vi "Vision_Processing_R_R6.vi"(0 "Current State":T1(ring)=enum."Normal - 5", 1 "Image Dst":T6=refnum, 2 "Inpute Image":T6=refnum, 3 "Startup Flag":bool, 5 "Current ROI Descriptor":T11={"Global Rectangle"=[0, 0, 320, 240], "Contours"=[{"ID"=enum."External", "Type"=12, "Coordinates"=[0, 0, 320, 240, 0]}]} {"Contours"."Type" items=["No Selection", "Point", "Line", "Rectangle", "Oval", "Polygon", "Freehand Region", "Annulus", "Unused2", "Unused3", "Broken Line", "Freehand Line", "Rotated Rectangle"]}, 6 "Avg Score - Last":dbl=802.5034383138021, 7 "error in (no error)":errorcluster, 8 "Current Settings":T9={"Curve Parameters"={"Extraction Mode"=1, "Edge Threshold"=150, "Edge Filter Size"=0, "Min Length"=25, "Row Search Step Size"=15, "Col Search Step Size"=15, "Max Endpoint Gap"=2, "Closed"=TRUE, "Subpixel"=TRUE}, "Match Mode"={"Rotation"=TRUE, "Scale"=TRUE, "Occlusion"=TRUE, "Reserved"=FALSE, "Reserved"=FALSE, "Reserved"=FALSE}, "Range Settings"=[{"Match Constraints"=0, "Min"=-5.0, "Max"=5.0}, {"Match Constraints"=1, "Min"=20.0, "Max"=150.0}, {"Match Constraints"=2, "Min"=0.0, "Max"=25.0}], "Number of Matches"=1, "Minimum Match Score"=800.0, "SubPixel Accuracy"=TRUE, "Adv. Geometric Match Options 2"=[{"Setup Data Item"=20, "Item Value"=0.0}, {"Setup Data Item"=22, "Item Value"=1.0}]} {"Curve Parameters"."Extraction Mode" items=["Normal", "Uniform Regions"]; "Curve Parameters"."Edge Filter Size" items=["Fine", "Normal", "Contour Tracing"]; "Curve Parameters"."Max Endpoint Gap" min=0; "Curve Parameters"."Col Search Step Size" min=1 max=255 step=1; "Curve Parameters"."Row Search Step Size" min=1 max=255 step=1; "Curve Parameters"."Min Length" min=0; "Curve Parameters"."Edge Threshold" min=1 max=350 step=1; "Range Settings"."Max" format="%.2f"; "Range Settings"."Min" format="%.2f"; "Range Settings"."Match Constraints" items=["Rotation Angle (degrees)", "Scale Factor (%)", "Occlusion (%)"]; "Adv. Geometric Match Options 2"."Setup Data Item" items=["Curve Extraction Mode", "Curve Edge Threshold", "Curve Edge Filter Size", "Min Curve Length", "Curve Row Search Step Size", "Curve Col Search Step Size", "Curve Max Endpoint Gap", "Extract Closed Curves", "Enable Subpixel Curve Extraction", "Enable Correlation Score", "Enable Subpixel Accuracy", "Subpixel Iterations", "Subpixel Tolerance", "Initial Match List Length", "Enable Target Template Curve Score", "Min Match Separation Distance", "Min Match Separation Angle", "Min Match Separation Scale", "Max Match Overlap", "Enable Coarse Result", "Enable Calibration Support", "Enable Contrast Reversal", "Search Strategy", "Refinement Match Factor", "Subpixel Match Factor"]}, 9 "Sub Beacon Search Enable":bool[](array[boolean])=[FALSE, FALSE, FALSE, FALSE, FALSE], 10 "History Data - IN":T5={"Valid Beacon History - in"=[FALSE, FALSE, FALSE, FALSE, FALSE, FALSE, FALSE, FALSE, FALSE, FALSE, FALSE, FALSE, FALSE, FALSE, FALSE, FALSE, FALSE, FALSE, FALSE, FALSE], "Valid Score History"=[916.1194458007812, 0.0, 921.171142578125, 952.2998657226562, 947.6416015625, 946.7607421875, 946.6710815429688, 913.2891235351562, 946.3783569335938, 946.1008911132812, 949.7362060546875, 948.7965087890625, 947.1905517578125, 948.5363159179688, 949.03466796875, 951.10986328125, 800.9814453125, 952.3334350585938, 926.0540161132812, 946.85888671875], "Valid Scale History"=[77.35153198242188, 0.0, 77.18988037109375, 76.20046997070312, 76.42532348632812, 76.47498321533203, 76.45317840576172, 77.11006927490234, 76.4490966796875, 76.39661407470703, 76.34481048583984, 76.36200714111328, 76.56851196289062, 76.3750228881836, 76.43797302246094, 76.20098876953125, 68.23258972167969, 76.18832397460938, 77.75858306884766, 76.44164276123047]} {"Valid Scale History" format="%#_13g"; "Valid Score History" format="%#_13g"}, 13 "Avg Scale - Last":dbl=73.9835688273112, 16 "History Size":i32=20) -> (11 "Avg Scale":dbl=73.9835688273112, 12 "Avg Score":dbl=802.5034383138021, 14 "Tracking Info":T2={"Tracking Coordinates"={"X"=0.0, "Y"=0.0}, "Current Valid"=FALSE, "Current State - Out"=enum."Normal - 5"}, 15 "Next Main ROI Descriptor":T3 {"Contours"."Type" items=["No Selection", "Point", "Line", "Rectangle", "Oval", "Polygon", "Freehand Region", "Annulus", "Unused2", "Unused3", "Broken Line", "Freehand Line", "Rotated Rectangle"]}, 17 "Beacon - Scales":sgl[](array[numeric])=[0.0, 0.0, 133.74268, 128.61499, 0.0], 18 "History Data - Out":T4={"Valid Beacon History\nOut"=[FALSE, FALSE, FALSE, FALSE, FALSE, FALSE, FALSE, FALSE, FALSE, FALSE, FALSE, FALSE, FALSE, FALSE, FALSE, FALSE, FALSE, FALSE, FALSE, FALSE], "Valid Score History\nOut"=[916.1194458007812, 0.0, 921.171142578125, 952.2998657226562, 947.6416015625, 946.7607421875, 946.6710815429688, 913.2891235351562, 946.3783569335938, 946.1008911132812, 949.7362060546875, 948.7965087890625, 947.1905517578125, 948.5363159179688, 949.03466796875, 951.10986328125, 800.9814453125, 952.3334350585938, 926.0540161132812, 946.85888671875], "Valid Scale History\nOut"=[77.35153198242188, 0.0, 77.18988037109375, 76.20046997070312, 76.42532348632812, 76.47498321533203, 76.45317840576172, 77.11006927490234, 76.4490966796875, 76.39661407470703, 76.34481048583984, 76.36200714111328, 76.56851196289062, 76.3750228881836, 76.43797302246094, 76.20098876953125, 68.23258972167969, 76.18832397460938, 77.75858306884766, 76.44164276123047]} {"Valid Scale History\nOut" format="%#_13g"; "Valid Score History\nOut" format="%#_13g"}, 19 "Y Coordinates":sgl[](array[numeric])=[0.0, 0.0, 133.74268, 128.61499, 0.0], 20 "Beacons Found":bool[](array[boolean])=[FALSE, FALSE, TRUE, TRUE, FALSE], 21 "X Coordinates":sgl[](array[numeric])=[0.0, 0.0, 162.26208, 213.98871, 0.0], 22 "Next State":T1(ring)=enum."Normal - 5", 23 "Lock Status":bool, 24 "Startup Flag - out":bool, 25 "New Settings":T9={"Curve Parameters"={"Extraction Mode"=1, "Edge Threshold"=150, "Edge Filter Size"=0, "Min Length"=25, "Row Search Step Size"=15, "Col Search Step Size"=15, "Max Endpoint Gap"=2, "Closed"=TRUE, "Subpixel"=TRUE}, "Match Mode"={"Rotation"=TRUE, "Scale"=TRUE, "Occlusion"=TRUE, "Reserved"=FALSE, "Reserved"=FALSE, "Reserved"=FALSE}, "Range Settings"=[{"Match Constraints"=0, "Min"=-5.0, "Max"=5.0}, {"Match Constraints"=1, "Min"=20.0, "Max"=150.0}, {"Match Constraints"=2, "Min"=0.0, "Max"=25.0}], "Number of Matches"=1, "Minimum Match Score"=800.0, "SubPixel Accuracy"=TRUE, "Adv. Geometric Match Options 2"=[{"Setup Data Item"=20, "Item Value"=0.0}, {"Setup Data Item"=22, "Item Value"=1.0}]} {"Curve Parameters"."Extraction Mode" items=["Normal", "Uniform Regions"]; "Curve Parameters"."Edge Filter Size" items=["Fine", "Normal", "Contour Tracing"]; "Curve Parameters"."Max Endpoint Gap" min=0; "Curve Parameters"."Col Search Step Size" min=1 max=255 step=1; "Curve Parameters"."Row Search Step Size" min=1 max=255 step=1; "Curve Parameters"."Min Length" min=0; "Curve Parameters"."Edge Threshold" min=1 max=350 step=1; "Range Settings"."Max" format="%.2f"; "Range Settings"."Min" format="%.2f"; "Range Settings"."Match Constraints" items=["Rotation Angle (degrees)", "Scale Factor (%)", "Occlusion (%)"]}, 27 "Right Image 2":T6(plugin-control))   [LabVIEW 2015]
uses:
  <vilib>/vision/Image Controls.llb/IMAQ Image.ctl
  <vilib>/vision/Pattern Matching.llb/IMAQ Curve Parameters.ctl
  <vilib>/vision/Pattern Matching.llb/IMAQ Match Range Setting.ctl
panel:
  in  "Sub - 4 - FIle Path":path=path "/home/lvuser/natinst/bin/BeaconTemplates/4_beacons_right.png"
  in  "3 / 2\nTransition Scale":sgl=100.0
  in  "Score\nCushion- tight":dbl=75.0
  in  "Main ROI Decay\nper Fail (Vertical)":i32=5
  in  "ROI_factor(Horiztonal) SCR":sgl=1.7
  in  "ROI_factor(vertical) SCR":sgl=1.5
  in  "Sub - 2 File Path":path=path "/home/lvuser/natinst/bin/BeaconTemplates/2_beacons_right.png"
  in  "Scale Decay \nFactor":dbl=0.5
  in  "Scale Decay \nFactor":dbl=5.0
  in  "Valid Treshold\nfor Lock":i16=3
  in  "Horiztonall Beacon \nCushion (pixels)":sgl=25.0
  out "New Min Score":dbl=800.0
  out "New Low Scale":dbl=20.0
  out "New high Scale":dbl=150.0
  in  "Absolute\nMinimum Score":dbl=700.0
  in  "Absolute\nMaximum Scale":dbl=300.0
  in  "Absolute\nMinimum Scale":dbl=10.0
  in  "Default No Lock\nSetting Values":T10={"Min Scale"=20.0, "Max Scale"=170.0, "Min Score"=800.0}
  in  "Score\nCushion":dbl=125.0
  in  "Scale \nCushion":dbl=7.0
  in  "5 / 4\nTransition Scale":sgl=78.0
  in  "4 / 3\nTransition Scale":sgl=85.0
  in  "Timeout \nThrehsold":i32=1000
  in  "Main ROI Decay\nper Fail (Horiztonal)":i32=25
  in  "ROI_factor(Horiztonal) LR":sgl=5.0
  in  "ROI_factor(vertical) LR":sgl=1.5
  in  "ROI_factor(vertical) SR":sgl=2.7
  in  "ROI_factor(Horiztonal) SR":sgl=2.0
  out "Current  Score":sgl=916.11945
  out "Current  Scale":sgl=77.35153
  in  "Fail Count - In":i32
  in  "Sub Beacon Template File Path - ARRAY":path[](array[path])=[path "/home/lvuser/natinst/bin/BeaconTemplates/Sub1.png", path "/home/lvuser/natinst/bin/BeaconTemplates/Sub2.png", path "/home/lvuser/natinst/bin/BeaconTemplates/Sub3.png", path "/home/lvuser/natinst/bin/BeaconTemplates/Sub4.png", path "/home/lvuser/natinst/bin/BeaconTemplates/Sub5.png"]
  in  "Sub - 3 - FIle Path":path=path "/home/lvuser/natinst/bin/BeaconTemplates/3_beacons_right.png"
  in  "Normal - 5 - File Path":path=path "/home/lvuser/natinst/bin/BeaconTemplates/5_beacons.png"
  # "INPUTS"
  # "FILE PATHS"
  # "CONFIG"
  # "OUTPUTS"
  # "************"
  # "Range"
  # "Range"
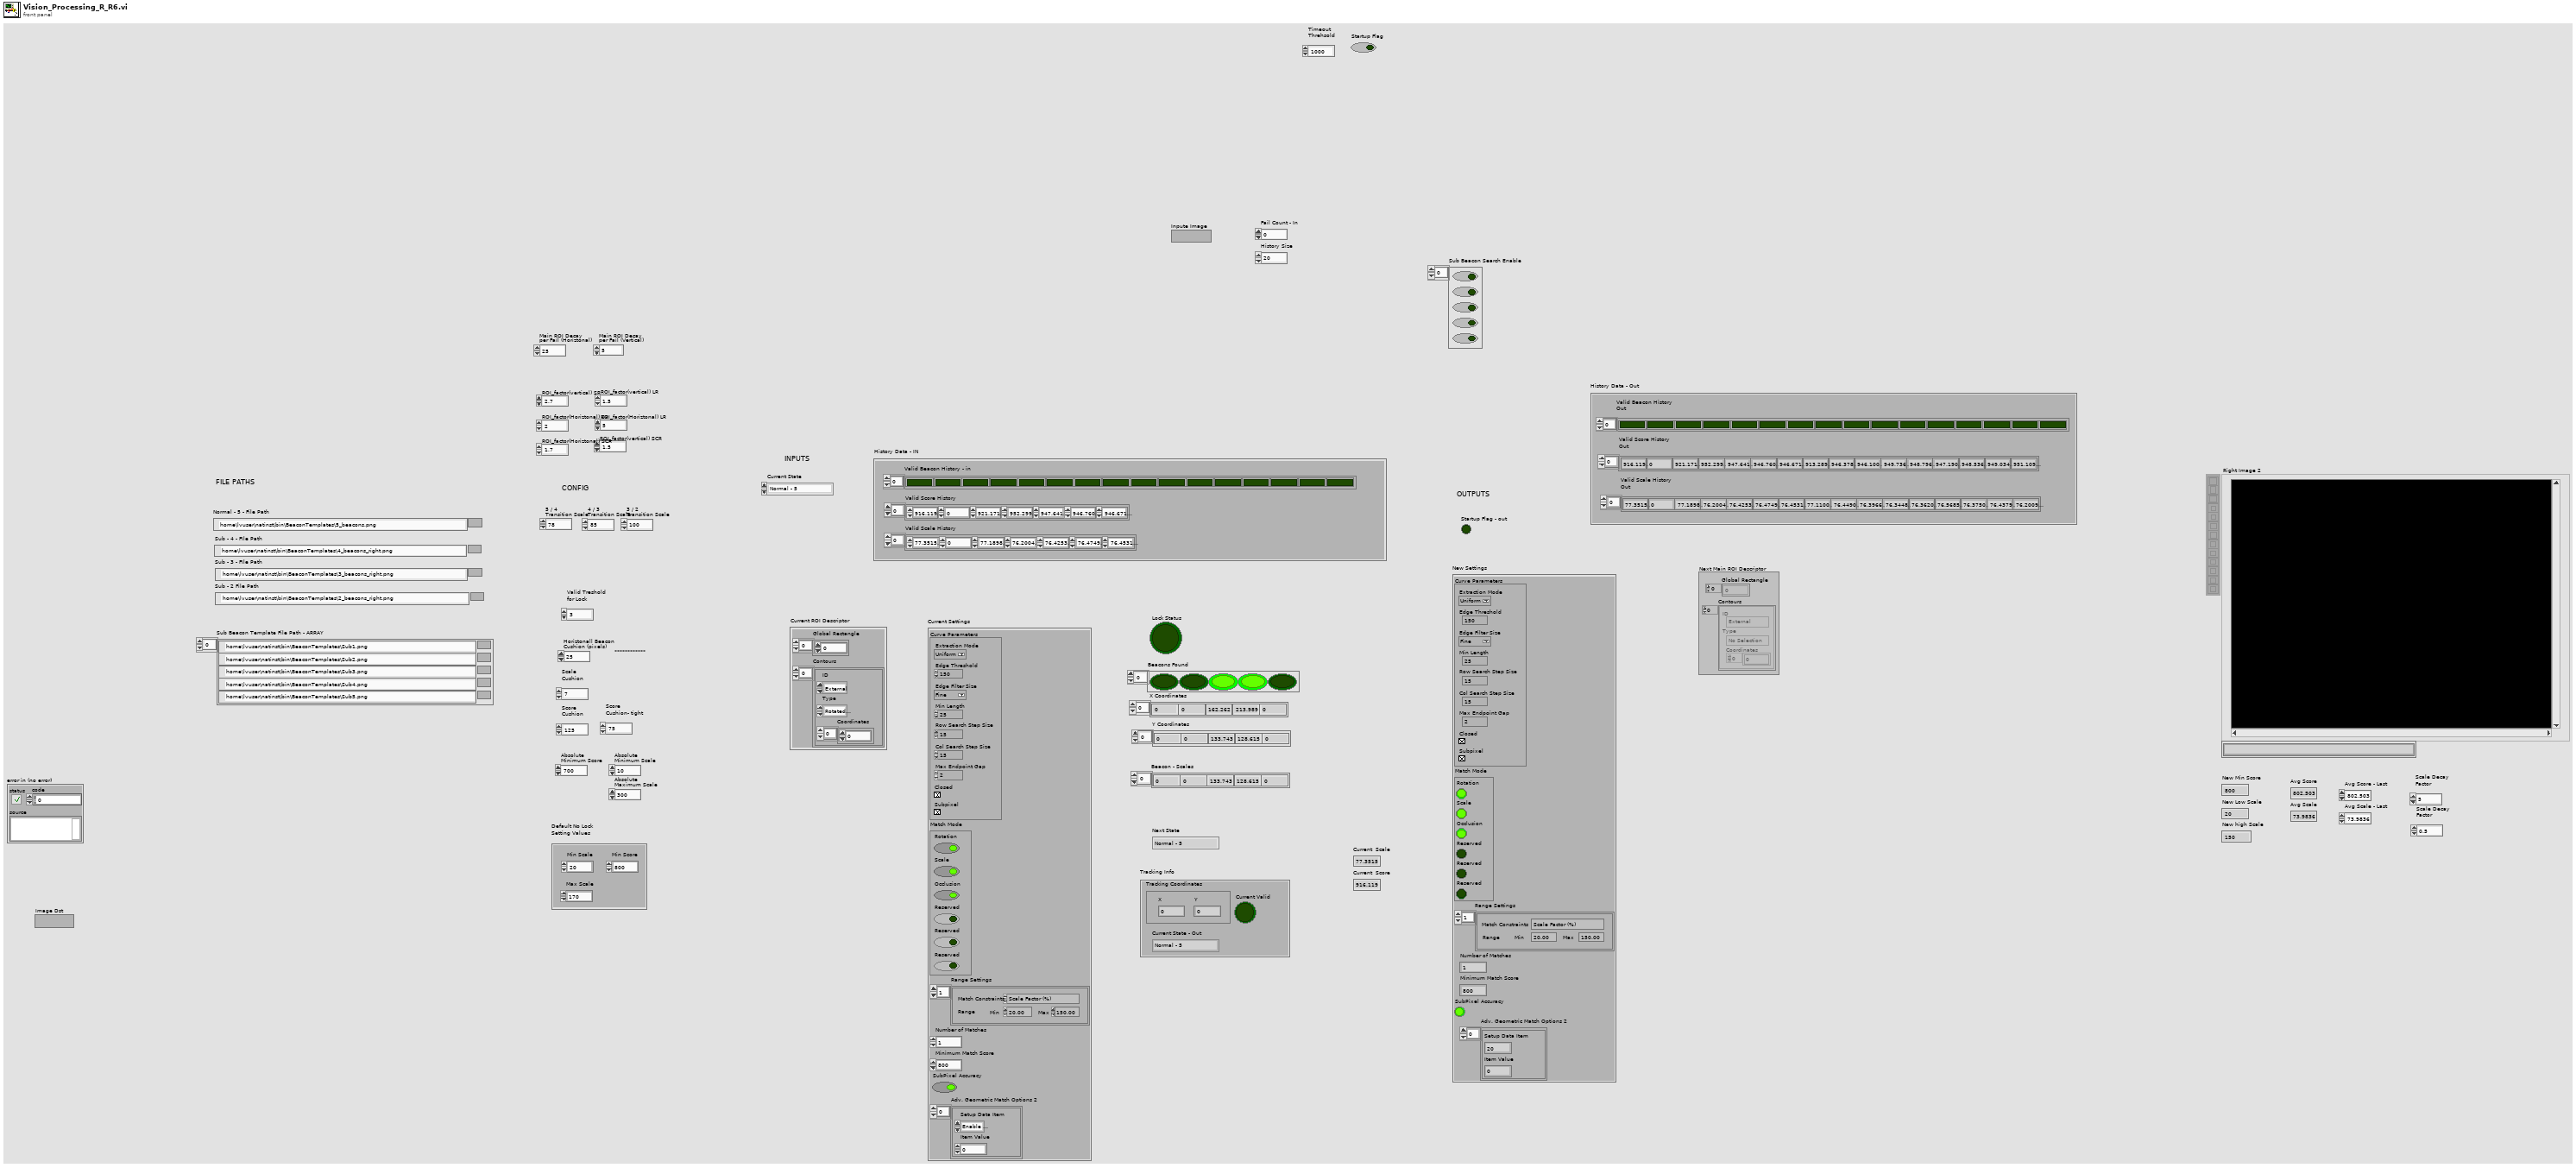
[diagram p1: front panel]
types:
  T1 = enum16{"Sub - 2", "Sub - 3", "Sub - 4", "Normal - 5"}
  T2 = cluster{"Tracking Coordinates":cluster{"X":dbl, "Y":dbl}, "Current Valid":bool, "Current State - Out":enum16{"Sub - 2", "Sub - 3", "Sub - 4", "Normal - 5"}}
  T3 = typedef "ROI Descriptor" = cluster{"Global Rectangle":i32[], "Contours":cluster{"ID":enum32{"External", "Internal"}, "Type":u32, "Coordinates":i32[]}[]}
  T4 = cluster{"Valid Beacon History\nOut":bool[], "Valid Score History\nOut":dbl[], "Valid Scale History\nOut":dbl[]}
  T5 = cluster{"Valid Beacon History - in":bool[], "Valid Score History":dbl[], "Valid Scale History":dbl[]}
  T6 = typedef "IMAQ Image.ctl" = refnum<image>
  T7 = typedef "IMAQ Curve Parameters.ctl" = cluster{"Extraction Mode":u32, "Edge Threshold":i32, "Edge Filter Size":u32, "Min Length":i32, "Row Search Step Size":i32, "Col Search Step Size":i32, "Max Endpoint Gap":i32, "Closed":bool, "Subpixel":bool}
  T8 = typedef "IMAQ Match Range Setting.ctl" = cluster{"Match Constraints":u32, "Min":dbl, "Max":dbl}
  T9 = cluster{"Curve Parameters":T7, "Match Mode":cluster{"Rotation":bool, "Scale":bool, "Occlusion":bool, "Reserved":bool, "Reserved":bool, "Reserved":bool}, "Range Settings":T8[], "Number of Matches":i32, "Minimum Match Score":sgl, "SubPixel Accuracy":bool, "Adv. Geometric Match Options 2":cluster{"Setup Data Item":u16, "Item Value":dbl}[]}
  T10 = cluster{"Min Scale":dbl, "Max Scale":dbl, "Min Score":dbl}
  T11 = cluster{"Global Rectangle":i32[], "Contours":cluster{"ID":enum32{"External", "Internal"}, "Type":u32, "Coordinates":i32[]}[]}
  T12 = typedef "IMAQ GM Match Report.ctl" = cluster{"Position":cluster{"x":sgl, "y":sgl}, "Angle":sgl, "Scale":sgl, "Score":sgl, "Bounding Box":cluster{"x":sgl, "y":sgl}[], "Contrast Reversed":bool, "Occlusion %":sgl, "Template Target Curve Score":sgl, "Target Template Curve Score":sgl, "Correlation Score":sgl}
  T13 = cluster{"Matches (Geometric Matching 1)[0]":T12, "Matches (Geometric Matching 1)[1]":T12, "Matches (Geometric Matching 1)[2]":T12, "Matches (Geometric Matching 1)[3]":T12, "Matches (Geometric Matching 1)[4]":T12, "Matches (Geometric Matching 1)[5]":T12, "Matches (Geometric Matching 1)[6]":T12, "Matches (Geometric Matching 1)[7]":T12, "Matches (Geometric Matching 1)[8]":T12}
  T14 = cluster{"Bounding Box[0]":cluster{"x":sgl, "y":sgl}, "Bounding Box[1]":cluster{"x":sgl, "y":sgl}, "Bounding Box[2]":cluster{"x":sgl, "y":sgl}, "Bounding Box[3]":cluster{"x":sgl, "y":sgl}, "Bounding Box[4]":cluster{"x":sgl, "y":sgl}, "Bounding Box[5]":cluster{"x":sgl, "y":sgl}, "Bounding Box[6]":cluster{"x":sgl, "y":sgl}, "Bounding Box[7]":cluster{"x":sgl, "y":sgl}, "Bounding Box[8]":cluster{"x":sgl, "y":sgl}}
  T15 = cluster{"Position":cluster{"x":sgl, "y":sgl}, bool, "Current State":enum16{"Sub - 2", "Sub - 3", "Sub - 4", "Normal - 5"}}
  T16 = typedef "IMAQ Rectangle" = cluster{"Left":i32, "Top":i32, "Right":i32, "Bottom":i32, "Rotation":dbl}
  T17 = cluster{"index":u32, "Min Scale":dbl, "Max Scale":dbl}
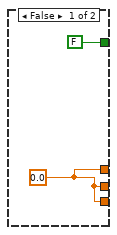
[diagram p2: hidden frame]
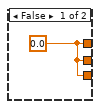
[diagram p3: hidden frame]
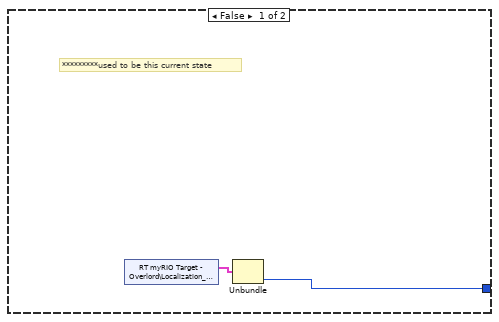
[diagram p7: hidden frame]
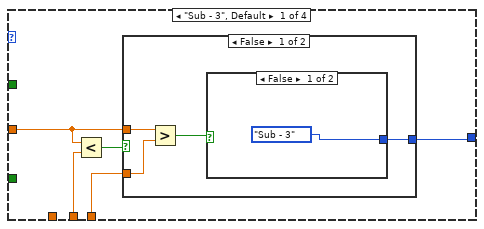
[diagram p8: hidden frame]
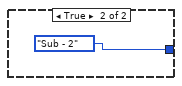
[diagram p9: hidden frame]
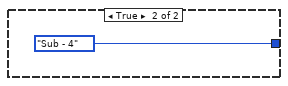
[diagram p10: hidden frame]
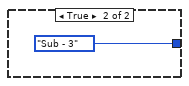
[diagram p11: hidden frame]
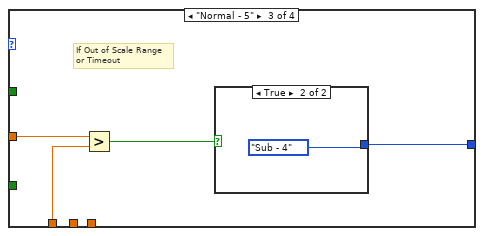
[diagram p12: hidden frame]
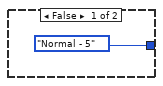
[diagram p13: hidden frame]
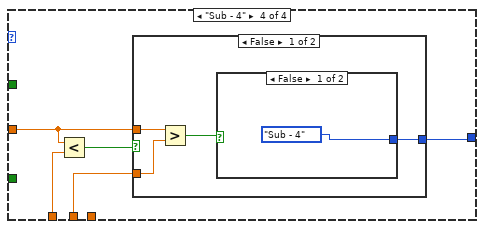
[diagram p14: hidden frame]
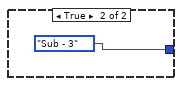
[diagram p15: hidden frame]
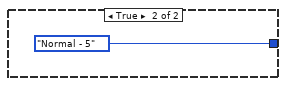
[diagram p16: hidden frame]
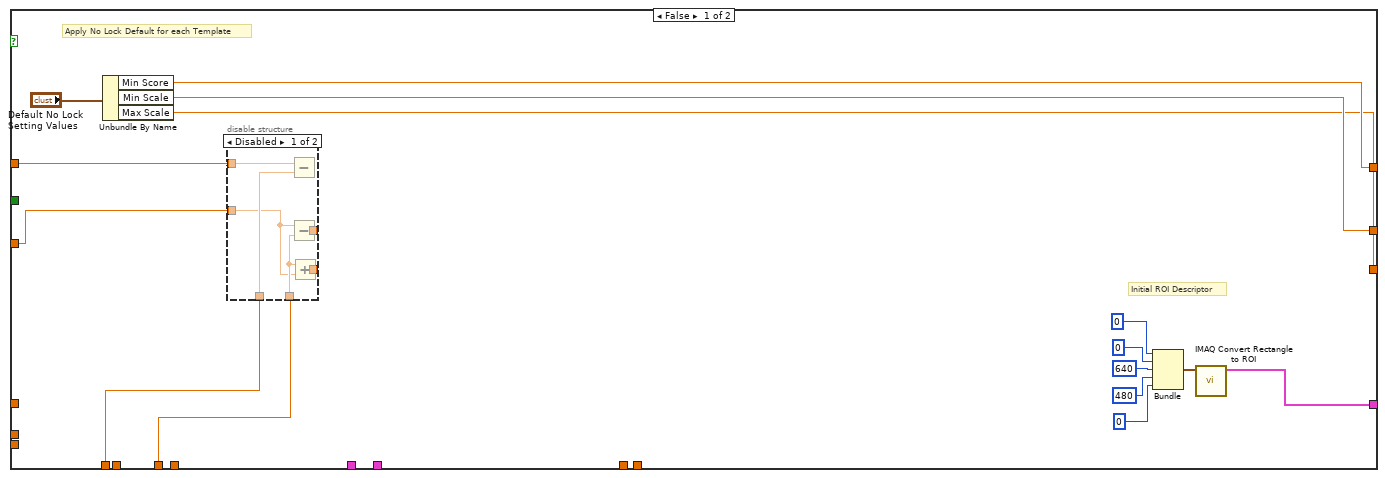
[diagram p18: hidden frame]
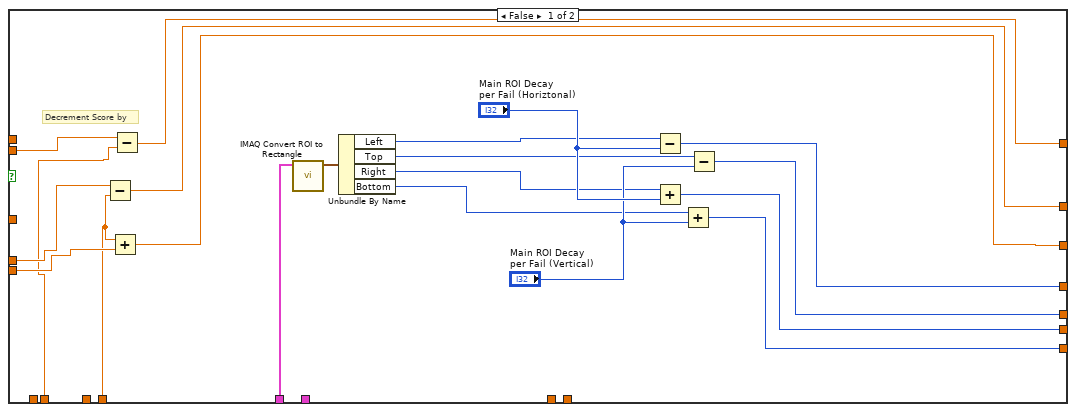
[diagram p20: hidden frame]
diagram:
  (unwired) enum16{"Short Range", "Long Range"}."Short Range"
  # "Next Settings"
  n1 = flat-sequence {
    tunnel: [w8] -> w3
    tunnel: [w7] -> w2
    tunnel: ["Image Dst"] -> w1
    tunnel: w3 -> [w131]
    tunnel: w2 -> [w129]
    tunnel: w1 -> [w130]
    frame #0 {
      # "APPLY FILTERING"
      n2 = call "Camera - Filtering"("Image In"="Inpute Image", "Image Dst"="Image Dst", "error in"="error in (no error)") -> ("Image Out"=w8:T6, "error out"=w7:errorcluster)  [unwired: 23 in]
    }
    frame #1 {
      w90 = u32 1 ("index")
      w111 = u8 5
      # "Start up Template"
      # "Image Lock"
      # "Current is Valid"
      # "Update Tracking Coordinates"
      # "CURRENT VALID"
      # "*************"
      # "Beacon - Y"
      # "Beacon - X"
      # "Beacons Found"
      # "Build ROI for Individual Beacons Based on Main Bounding Box"
      # "Starting X Lower Bound"
      # "Length of\nIndividual Beacon ROI"
      # "Length of Bounding Box"
      # "Choose ROI Factor based on Next State"
      # "Current Match"
      # "Current ROI"
      # "Image Lock"
      # "Force SR on Startup"
      # "Valid History"
      # "Draw ROI and stuff on outputi mage"
      # "Pull Down Startup IF Already True and Lock\nOtherwise don't update"
      # "Next Settings"
      # "Apply Limits to Settings"
      # "Scale"
      # "Min Score"
      # "Lower Scale"
      # "Upper Scale"
      # "Current Settings"
      # "Current Min\n& Max Scale"
      # "Current Valid"
      # "Update Search Settings"
      # "Update Template State"
      # "Calculate Average Scale/Score"
      # "max avg"
      # "Min Required to use avarage"
      # "Valid  Ccount\n(up to 3)"
      # "****# of previous in history that must be true\nin order for position to be considered \"locked\""
      # "Update Shift Arrays"
      # "# of Beacons Found to be valid"
      # "# of beacons"
      # "Matches"
      # "image out"
      n3 = Select(t=T1."Normal - 5", s="Startup Flag", f="Current State") -> (s? t:f=w12:T1)
      n4 = case shown="\"Sub - 2\"" w12 {
        tunnel: w131 -> [w408 w440 w471 w506]
        tunnel: w130 -> [w407 w439 w470 w505]
        tunnel: "Current ROI Descriptor" -> [w406 w438 w468 w504]
        tunnel: "Current Settings" -> [w405 w437 w467 w503]
        tunnel: [w401 w433 w464 w499] -> w49
        tunnel: [w400 w432 w465 w498] -> w70
        tunnel: [w398 w430 w466 w496] -> w120
        tunnel: w129 -> [_ _ w469 w495]
        tunnel: "Sub Beacon Search Enable" -> [w399 w431 w472 w494]
        tunnel: [sgl 3.0 ("y") sgl 2.0 ("y") 4.0 sgl 5.0 ("y")] -> w127
        tunnel: [w396 w428 w462 w492] -> w126
        tunnel: [2 1 3 4] -> w121
        frame "Sub - 3" {
          n5 = call "Short Range 2"("Image In"=w408, "Image Dst"=w407, "ROI Descriptor (Geometric Matching 1)"=w406, "Settings (Geometric Matching 1)"=w405, "Template File Path (Geometric Matching 1)"="Sub - 3 - FIle Path") -> ("Image Out"=w400:T6, "Matches (Geometric Matching 1)"=w401:T12[], "Number of Matches (Geometric Matching 1)"=w402:i32, "error out"=w396:errorcluster)  [unwired: 19 in]
          n6 = Equal?(x=w402, y=1) -> (x = y?=w403:bool)
          n7 = case shown="True" w403 {
            tunnel: w399 -> [w416 w419]
            tunnel: [w409 w420] -> w398
            frame False {
              w410 = FALSE
              # "F"
              # "No Main Found,\nDon't Search any Subs"
              n8 = Replace Array Subset(array=w416, new element #1=w410, index #1=0 ("y"), new element #2=w410, index #2=1 ("y"), new element #3=w410, index #3=2 ("y"), new element #4=w410, index #4=3 ("y"), new element #5=w410, index #5=4 ("y")) -> (w409:bool[])
            }
            frame True {
              w418 = TRUE
              w417 = FALSE
              n9 = Replace Array Subset(array=w419, new element #1=w417, index #1=0 ("y"), new element #2=w417, index #2=1 ("y"), new element #3=w418, index #3=2 ("y"), new element #4=w418, index #4=3 ("y"), new element #5=w418, index #5=4 ("y")) -> (w420:bool[])
            }
          }
        }
        frame "Sub - 2" {
          n10 = call "Short Range"("Image In"=w440, "Image Dst"=w439, "ROI Descriptor (Geometric Matching 1)"=w438, "Settings (Geometric Matching 1)"=w437, "Template File Path (Geometric Matching 1)"="Sub - 2 File Path") -> ("Image Out"=w432:T6, "Matches (Geometric Matching 1)"=w433:T12[], "Number of Matches (Geometric Matching 1)"=w434:i32, "error out"=w428:errorcluster)  [unwired: 19 in]
          n11 = Equal?(x=w434, y=1) -> (x = y?=w435:bool)
          n12 = case shown="True" w435 {
            tunnel: w431 -> [w448 w451]
            tunnel: [w441 w452] -> w430
            frame False {
              w442 = FALSE
              # "F"
              # "No Main Found,\nDon't Search any Subs"
              n13 = Replace Array Subset(array=w448, new element #1=w442, index #1=0 ("y"), new element #2=w442, index #2=1 ("y"), new element #3=w442, index #3=2 ("y"), new element #4=w442, index #4=3 ("y"), new element #5=w442, index #5=4 ("y")) -> (w441:bool[])
            }
            frame True {
              w450 = TRUE
              w449 = FALSE
              # "Search for specific Beacons"
              n14 = Replace Array Subset(array=w451, new element #1=w449, index #1=0 ("y"), new element #2=w449, index #2=1 ("y"), new element #3=w449, index #3=2 ("y"), new element #4=w450, index #4=3 ("y"), new element #5=w450, index #5=4 ("y")) -> (w452:bool[])
            }
          }
        }
        frame "Sub - 4" {
          # "**Make sure this selects the \nappropriate beacons to search for!!"
          n15 = call "Dumping Range"("Image In"=w471, "Image Dst"=w470, "ROI Descriptor (Geometric Matching 1)"=w468, "Settings (Geometric Matching 1)"=w467, "Template File Path (Geometric Matching 1)"="Sub - 4 - FIle Path", "error in"=w469) -> ("Image Out"=w465:T6, "Matches (Geometric Matching 1)"=w464:T12[], "Number of Matches (Geometric Matching 1)"=w461:i32, "error out"=w462:errorcluster)  [unwired: 18 in]
          n16 = Equal?(x=w461, y=1) -> (x = y?=w459:bool)
          n17 = case shown="True" w459 {
            tunnel: w472 -> [w481 w484]
            tunnel: [w474 w485] -> w466
            frame False {
              w475 = FALSE
              # "F"
              # "No Main Found,\nDon't Search any Subs"
              n18 = Replace Array Subset(array=w481, new element #1=w475, index #1=0 ("y"), new element #2=w475, index #2=1 ("y"), new element #3=w475, index #3=2 ("y"), new element #4=w475, index #4=3 ("y"), new element #5=w475, index #5=4 ("y")) -> (w474:bool[])
            }
            frame True {
              w483 = TRUE
              n19 = Replace Array Subset(array=w484, new element #1=FALSE, index #1=0 ("y"), new element #2=w483, index #2=1 ("y"), new element #3=w483, index #3=2 ("y"), new element #4=w483, index #4=3 ("y"), new element #5=w483, index #5=4 ("y")) -> (w485:bool[])
            }
          }
        }
        frame "Normal - 5" {
          n20 = call "Long Range"("Image In"=w506, "Image Dst"=w505, "ROI Descriptor (Geometric Matching 1)"=w504, "Settings (Geometric Matching 1)"=w503, "Template File Path (Geometric Matching 1)"="Normal - 5 - File Path", "error in"=w495) -> ("Image Out"=w498:T6, "Matches (Geometric Matching 1)"=w499:T12[], "Number of Matches (Geometric Matching 1)"=w501:i32, "error out"=w492:errorcluster)  [unwired: 18 in]
          n21 = Equal?(x=w501, y=1) -> (x = y?=w497:bool)
          n22 = case shown="True" w497 {
            tunnel: w494 -> [w514 w516]
            tunnel: [w507 w515] -> w496
            frame False {
              w508 = FALSE
              # "F"
              # "No Main Found,\nDon't Search any Subs"
              n23 = Replace Array Subset(array=w514, new element #1=w508, index #1=0 ("y"), new element #2=w508, index #2=1 ("y"), new element #3=w508, index #3=2 ("y"), new element #4=w508, index #4=3 ("y"), new element #5=w508, index #5=4 ("y")) -> (w507:bool[])
            }
            frame True {
              w517 = TRUE
              # "T"
              # "Search for ALL Beacons"
              n24 = Replace Array Subset(array=w516, new element #1=w517, index #1=0 ("y"), new element #2=w517, index #2=1 ("y"), new element #3=w517, index #3=2 ("y"), new element #4=w517, index #4=3 ("y"), new element #5=w517, index #5=4 ("y")) -> (w515:bool[])
            }
          }
        }
      }
      n25 = Array To Cluster(array=w49) -> (cluster=w39:T13)
      n26 = Unbundle By Name(w39) -> ("Matches (Geometric Matching 1)[0].Position"=w14:cluster{"x":sgl, "y":sgl}, "Matches (Geometric Matching 1)[0].Bounding Box"=w37:cluster{"x":sgl, "y":sgl}[], "Matches (Geometric Matching 1)[0].Scale"=w69:sgl, "Matches (Geometric Matching 1)[0].Score"=w81:sgl)
      "Current  Scale" <- w69
      "Current  Score" <- w81
      n27 = Array To Cluster(array=w37) -> (cluster=w38:T14)
      n28 = Unbundle By Name(w38) -> ("Bounding Box[0].x"=w28:sgl, "Bounding Box[0].y"=w27:sgl, "Bounding Box[2].x"=w26:sgl, "Bounding Box[2].y"=w25:sgl)
      n29 = Bundle("x"=w28, "y"=w27, "x"=w26, "y"=w25) -> (w23:cluster{"x":sgl, "y":sgl, "x":sgl, "y":sgl})  [unwired: 1 in]
      n30 = call "IMAQ Overlay Rectangle"("Rectangle"=w23, "Image"=w70) -> ("Image Out"=w24:T6)  [unwired: 8 in, 1 out]
      n31 = Subtract(x=w26, y=w28) -> (x-y=w32:sgl)
      n32 = Divide(x=w32, y=w127) -> (x/y=w34:dbl)
      n33 = Multiply(x="Horiztonall Beacon \nCushion (pixels)", y=w69) -> (x*y=w22:sgl)
      n34 = Divide(x=w22, y=sgl 100.0) -> (x/y=w19:sgl)
      n35 = Subtract(x=w27, y=w19) -> (x-y=w35:sgl)
      n36 = Add(x=w19, y=w25) -> (x+y=w36:sgl)
      n37 = for {
        N: 5 -> [_]
        tunnel: w120 -> [w174] mode=indexing
        shift-right: [w168] -> _
        shift-left: w28 -> [w173]
        tunnel: w34 -> [w172]
        tunnel: w35 -> [w165]
        tunnel: w36 -> [w164]
        tunnel: [w171] -> w30 mode=indexing
        tunnel: w19 -> [w166]
        # "Divide Bounding Box"
        # "Upper Bound of Current is\nLower Bound for Next"
        n38 = case shown="True" w174 {
          tunnel: w173 -> [w175 w176]
          tunnel: w172 -> [_ w178]
          tunnel: [w175 w177] -> w168
          tunnel: [w175 w176] -> w170
          frame False {
            # "Don't Care"
          }
          frame True {
            # "X Lower Bound"
            n39 = Add(x=w176, y=w178) -> (x+y=w177:dbl)
          }
        }
        n40 = Subtract(x=w170, y=w166) -> (x-y=w169:dbl)
        n41 = Add(x=w168, y=w166) -> (x+y=w167:dbl)
        n42 = call "Bound_RO_R_R0I.vi"("Bottom Right - Y"=w164, "Right - X"=w167, "Top Left - Y"=w165, "Top  Left - x"=w169) -> ("ROI Descriptor"=w171:T3)  [unwired: 7 in]
      }
      n43 = for {
        N: 5 -> [_]
        tunnel: w70 -> [w143]
        tunnel: w126 -> [w142]
        tunnel: w30 -> [w135] mode=indexing
        tunnel: "Sub Beacon Template File Path - ARRAY" -> [w141] mode=indexing
        tunnel: [w140] -> w125 mode=indexing
        tunnel: [w139] -> w124 mode=indexing
        tunnel: [w138] -> w112 mode=indexing
        tunnel: w120 -> [w137] mode=indexing
        tunnel: "Current Settings" -> [w136]
        shift-right: [w133] -> w71
        shift-left: w24 -> [w134]
        tunnel: [w132] -> w60 mode=indexing
        n44 = case shown="True" w137 {
          tunnel: w143 -> [_ w157]
          tunnel: w142 -> [_ w156]
          tunnel: w135 -> [_ w155]
          tunnel: w141 -> [_ w154]
          tunnel: [w144 w150] -> w140
          tunnel: [w144 w149] -> w139
          tunnel: [FALSE w148] -> w138
          tunnel: w136 -> [_ w147]
          tunnel: [w144 w146] -> w132
          frame False {
            w144 = sgl 0.0 ("x")
          }
          frame True {
            n45 = call "Sub Beacon Pattern Match"("Image In"=w157, "ROI Descriptor (Geometric Matching 1)"=w155, "Settings (Geometric Matching 1)"=w147, "Template File Path (Geometric Matching 1)"=w154, "error in"=w156) -> ("Matches (Geometric Matching 1)"=w151:T12[], "Number of Matches (Geometric Matching 1)"=w152:i32)  [unwired: 19 in, 2 out]
            n46 = Equal?(x=w152, y=1) -> (x = y?=w148:bool)
            n47 = case shown="True" w148 {
              tunnel: w151 -> [_ w162]
              tunnel: [w158 w161] -> w150
              tunnel: [w158 w160] -> w149
              tunnel: [w158 w159] -> w146
              frame False {
                w158 = sgl 0.0 ("x")
              }
              frame True {
                n48 = Array To Cluster(array=w162) -> (cluster=w163:T13)
                n49 = Unbundle By Name(w163) -> ("Matches (Geometric Matching 1)[0].Position.x"=w161:sgl, "Matches (Geometric Matching 1)[0].Position.y"=w160:sgl, "Matches (Geometric Matching 1)[0].Scale"=w159:sgl)
              }
            }
          }
        }
        n50 = call "IMAQ Overlay ROI"("ROI Descriptor"=w135, "Image"=w134) -> ("Image Out"=w133:T6)  [unwired: 8 in, 1 out]
      }
      "Beacons Found" <- w112
      "X Coordinates" <- w125
      "Y Coordinates" <- w124
      "Beacon - Scales" <- w60
      n51 = Boolean To (0,1)(Boolean=w112) -> (0, 1=w122:i16[])
      n52 = Add Array Elements(numeric array=w122) -> (sum=w123:i16)
      n53 = Greater Or Equal?(x=w123, y=w121) -> (x >= y?=w13:bool)
      n54 = case shown="False" w13 {
        tunnel: "Fail Count - In" -> [w392 _]
        tunnel: [w391 u16 0] -> w104
        frame False {
          n55 = Increment(x=w392) -> (x+1=w391:i32)
        }
        frame True {
          # "reset fail count"
        }
      }
      n56 = Unbundle By Name("History Data - IN") -> ("Valid Beacon History - in"=w67:bool[], "Valid Score History"=w66:dbl[], "Valid Scale History"=w65:dbl[])
      n57 = Greater?(x=w104, y="Timeout \nThrehsold") -> (0:w16:bool)
      n58 = Decrement(x="History Size") -> (x-1=w118:i32)
      n59 = for {
        N: "History Size" -> [_]
        shift-right: [w369] -> w64
        shift-left: w67 -> [w357]
        tunnel: w118 -> [w365]
        shift-right: [w362] -> w63
        shift-left: w66 -> [w364]
        shift-right: [w361] -> w62
        shift-left: w65 -> [w363]
        tunnel: w81 -> [w360]
        tunnel: w69 -> [w359]
        tunnel: w13 -> [w358]
        i -> [w368]
        # "Reverse Index"
        n60 = Subtract(x=w365, y=w368) -> (x-y=w366:i32)
        n61 = Equal To 0?(x=w366) -> (x = 0?=w367:bool)
        n62 = case shown="True" w367 {
          tunnel: w366 -> [w370 w389]
          tunnel: w357 -> [w380 w382]
          tunnel: [w378 w381] -> w369
          tunnel: w358 -> [_ w390]
          tunnel: w364 -> [w375 w388]
          tunnel: w363 -> [w374 w387]
          tunnel: [w373 w385] -> w362
          tunnel: [w372 w386] -> w361
          tunnel: w360 -> [_ w384]
          tunnel: w359 -> [_ w383]
          frame False {
            # "Shift Old"
            n63 = Decrement(x=w370) -> (x-1=w371:i32)
            n64 = Index Array(array=w380, index=w371) -> (element=w379:bool)
            n65 = Index Array(array=w375, index=w371) -> (element=w377:dbl)
            n66 = Index Array(array=w374, index=w371) -> (element=w376:dbl)
            n67 = Replace Array Subset(array=w380, new element=w379, index=w370) -> (w378:bool[])
            n68 = Replace Array Subset(array=w375, new element=w377, index=w370) -> (w373:dbl[])
            n69 = Replace Array Subset(array=w374, new element=w376, index=w370) -> (w372:dbl[])
          }
          frame True {
            # "Scale"
            # "Score"
            # "Valid"
            # "insert New"
            n70 = Replace Array Subset(array=w388, new element=w384, index=w389) -> (w385:dbl[])
            n71 = Replace Array Subset(array=w387, new element=w383, index=w389) -> (w386:dbl[])
            n72 = Replace Array Subset(array=w382, new element=w390, index=w389) -> (w381:bool[])
          }
        }
      }
      n73 = Boolean To (0,1)(Boolean=w64) -> (0, 1=w116:i16[])
      n74 = Bundle("Valid Beacon History - in"=w64, "Valid Score History"=w63, "Valid Scale History"=w62) -> (→"History Data - Out":T5)  [unwired: 1 in]
      n75 = Add Array Elements(numeric array=w116) -> (sum=w117:i16)
      n76 = Greater Or Equal?(x=w117, y="Valid Treshold\nfor Lock") -> (x >= y?=w82:bool)
      "Lock Status" <- w82
      n77 = Initialize Array(u8 0, w111) -> (w114:u8[])
      n78 = while {
        shift-right: [w340] -> w109
        shift-left: w114 -> [w342]
        tunnel: w64 -> [w348] mode=indexing
        shift-right: [w346] -> w107
        shift-left: u8 0 -> [w349]
        tunnel: "History Size" -> [w347]
        tunnel: w111 -> [w339]
        i -> [w341]
        stop <- w343 stop-if-true
        # "Grab Last 2 Valid Indexes"
        n79 = case shown="True" w348 {
          tunnel: w349 -> [w351 w353]
          tunnel: [w351 w356] -> w346
          tunnel: w342 -> [w350 w355]
          tunnel: w341 -> [_ w354]
          tunnel: [w350 w352] -> w340
          frame False {
          }
          frame True {
            # "Update Index\nto use"
            # "Increment\nValid Count"
            n80 = Replace Array Subset(array=w355, new element=w354, index=w353) -> (w352:u8[])
            n81 = Increment(x=w353) -> (x+1=w356:u8)
          }
        }
        n82 = Greater?(x=w341, y=w347) -> (0:w344:bool)
        n83 = Greater Or Equal?(x=w346, y=w339) -> (x >= y?=w345:bool)
        n84 = Or(x=w345, y=w344) -> (x .or. y?=w343:bool)
      }
      n85 = Greater?(x=w107, y=u8 2) -> (0:w108:bool)
      n86 = case shown="False" w108 {
        tunnel: w107 -> [_ w323]
        tunnel: w109 -> [_ w329]
        tunnel: w63 -> [_ w328]
        tunnel: w62 -> [_ w327]
        tunnel: ["Avg Score - Last" w321] -> w78
        tunnel: ["Avg Scale - Last" w320] -> w79
        frame False {
        }
        frame True {
          w326 = 0.0
          n87 = for {
            N: w323 -> [_]
            tunnel: w329 -> [w336] mode=indexing
            tunnel: w328 -> [w338]
            tunnel: w327 -> [w337]
            shift-right: [w334] -> w325
            shift-left: w326 -> [w332]
            shift-right: [w335] -> w324
            shift-left: w326 -> [w331]
            # "Fetch Last Valid Values"
            n88 = Index Array(array=w338, index=w336) -> (element=w333:dbl)
            n89 = Index Array(array=w337, index=w336) -> (element=w330:dbl)
            n90 = Add(x=w333, y=w332) -> (x+y=w334:dbl)
            n91 = Add(x=w330, y=w331) -> (x+y=w335:dbl)
          }
          n92 = To Double Precision Float(number=w323) -> (double precision float=w322:dbl)
          n93 = Divide(x=w325, y=w322) -> (x/y=w321:dbl)
          n94 = Divide(x=w324, y=w322) -> (x/y=w320:dbl)
        }
      }
      "Avg Score" <- w78
      "Avg Scale" <- w79
      n95 = Bundle("Position"=w14, w13, "Current State"=w12) -> (→"Tracking Info":T15)  [unwired: 1 in]
      n96 = case shown="True" w82 {
        tunnel: w16 -> [_ w193]
        tunnel: "4 / 3\nTransition Scale" -> [_ w192]
        tunnel: "5 / 4\nTransition Scale" -> [_ w191]
        tunnel: w79 -> [_ w190]
        tunnel: w82 -> [_ w189]
        tunnel: [w185 w188] -> w10
        tunnel: "3 / 2\nTransition Scale" -> [_ w187]
        frame False {
          # "*********used to be this current state"
          n97 = shared-variable "RT myRIO Target - Overlord\\Localization_Variables_r0.lvlib\\Info - Left"() -> (w186:T2)  [unwired: 1 in, 1 out]
          n98 = Unbundle(w186) -> ("Current State - Out"=w185:T1)  [unwired: 2 out]
        }
        frame True {
          # "Timeout"
          n99 = local read "Current State"() -> (w194:T1)
          n100 = case shown="\"Sub - 2\"" w194 {
            tunnel: w189 -> [_ _ _ _]
            tunnel: w190 -> [w198 w210 w215 w221]
            tunnel: w193 -> [_ _ _ _]
            tunnel: w192 -> [w199 _ _ w220]
            tunnel: w191 -> [_ _ w214 w223]
            tunnel: [w195 w207 w213 w219] -> w188
            tunnel: w187 -> [w196 w209 _ _]
            frame "Sub - 3", Default {
              n101 = Less?(x=w198, y=w199) -> (x < y?=w197:bool)
              n102 = case shown="False" w197 {
                tunnel: w198 -> [w203 _]
                tunnel: [w200 T1."Sub - 4"] -> w195
                tunnel: w196 -> [w202 _]
                frame False {
                  n103 = Greater?(x=w203, y=w202) -> (0:w201:bool)
                  n104 = case shown="False" w201 {
                    tunnel: [T1."Sub - 3" T1."Sub - 2"] -> w200
                    frame False {
                    }
                    frame True {
                    }
                  }
                }
                frame True {
                }
              }
            }
            frame "Sub - 2" {
              n105 = Less?(x=w210, y=w209) -> (x < y?=w208:bool)
              n106 = case shown="False" w208 {
                tunnel: [T1."Sub - 2" T1."Sub - 3"] -> w207
                frame False {
                }
                frame True {
                }
              }
            }
            frame "Normal - 5" {
              # "If Out of Scale Range\nor Timeout"
              n107 = Greater?(x=w215, y=w214) -> (0:w216:bool)
              n108 = case shown="True" w216 {
                tunnel: [T1."Normal - 5" T1."Sub - 4"] -> w213
                frame False {
                }
                frame True {
                }
              }
            }
            frame "Sub - 4" {
              n109 = Less?(x=w221, y=w223) -> (x < y?=w222:bool)
              n110 = case shown="False" w222 {
                tunnel: w221 -> [w227 _]
                tunnel: [w224 T1."Normal - 5"] -> w219
                tunnel: w220 -> [w226 _]
                frame False {
                  n111 = Greater?(x=w227, y=w226) -> (0:w225:bool)
                  n112 = case shown="False" w225 {
                    tunnel: [T1."Sub - 4" T1."Sub - 3"] -> w224
                    frame False {
                    }
                    frame True {
                    }
                  }
                }
                frame True {
                }
              }
            }
          }
        }
      }
      "Next State" <- w10
      n113 = Unbundle By Name("Current Settings") -> ("Minimum Match Score"=w101:sgl, "Range Settings"=w87:T8[])
      n114 = case shown="\"Sub - 4\", Default" w10 {
        tunnel: "ROI_factor(vertical) SR" -> [_ _ w184]
        tunnel: "ROI_factor(Horiztonal) SR" -> [_ _ w183]
        tunnel: "ROI_factor(vertical) LR" -> [_ w182 _]
        tunnel: "ROI_factor(Horiztonal) LR" -> [_ w181 _]
        tunnel: "ROI_factor(vertical) SCR" -> [w180 _ _]
        tunnel: "ROI_factor(Horiztonal) SCR" -> [w179 _ _]
        tunnel: [w180 w182 w184] -> w42
        tunnel: [w179 w181 w183] -> w41
        frame "Sub - 2" {
        }
        frame "Sub - 4", Default {
        }
        frame "Sub - 3" {
        }
      }
      n115 = Index Array(array=w87, index=u32 1) -> (element=w100:T8)
      n116 = Unbundle(w100) -> ("Min"=w98:dbl, "Max"=w97:dbl)  [unwired: 1 out]
      n117 = case shown="True" w82 {
        tunnel: w13 -> [_ w275]
        tunnel: w78 -> [w244 w274]
        tunnel: w79 -> [w243 w273]
        tunnel: w101 -> [_ w272]
        tunnel: w98 -> [_ w271]
        tunnel: w97 -> [_ w270]
        tunnel: [w242 w261] -> w88
        tunnel: [w241 w260] -> w53
        tunnel: [w240 w259] -> w54
        tunnel: "Scale \nCushion" -> [w246 w269]
        tunnel: "Score\nCushion" -> [w245 w268]
        tunnel: "Scale Decay \nFactor" -> [_ w267]
        tunnel: "Scale Decay \nFactor" -> [_ w266]
        tunnel: "Current ROI Descriptor" -> [_ w262]
        tunnel: w49 -> [_ w263]
        tunnel: w42 -> [_ w265]
        tunnel: w41 -> [_ w264]
        tunnel: [w233 w258] -> w40
        frame False {
          # "Initial ROI Descriptor"
          # "Apply No Lock Default for each Template"
          n118 = Unbundle By Name("Default No Lock\nSetting Values") -> ("Min Score"=w242:dbl, "Min Scale"=w241:dbl, "Max Scale"=w240:dbl)
          n119 = disable-structure shown="Disabled" {
            disable-tunnel: [w253 _] -> _
            disable-tunnel: [w252 _] -> _
            disable-tunnel: w246 -> [w251 _]
            disable-tunnel: w245 -> [w250 _]
            disable-tunnel: w244 -> [w249 _]
            disable-tunnel: w243 -> [w248 _]
            frame Disabled {
              n120 = Subtract(x=w249, y=w250) -> ()  [unwired: 1 out]
              n121 = Subtract(x=w248, y=w251) -> (x-y=w253:dbl)
              n122 = Add(x=w251, y=w248) -> (x+y=w252:dbl)
            }
            frame Enabled {
            }
          }
          n123 = Bundle(0, 0, 640, 480, 0) -> (w239:cluster{i32, i32, i32, i32, i32})  [unwired: 1 in]
          n124 = call "IMAQ Convert Rectangle to ROI"("Rectangle"=w239) -> ("ROI Descriptor"=w233:T3)  [unwired: 8 in, 1 out]
        }
        frame True {
          # "Apply Limits to ROI"
          n125 = case shown="True" w275 {
            tunnel: w274 -> [_ w317]
            tunnel: [w290 w313] -> w261
            tunnel: w273 -> [_ w316]
            tunnel: [w289 w312] -> w260
            tunnel: [w288 w311] -> w259
            tunnel: w271 -> [w295 _]
            tunnel: w270 -> [w294 _]
            tunnel: w272 -> [w293 _]
            tunnel: w269 -> [_ w315]
            tunnel: w268 -> [_ w314]
            tunnel: w267 -> [w292 _]
            tunnel: w266 -> [w291 _]
            tunnel: w265 -> [_ w302]
            tunnel: w264 -> [_ w301]
            tunnel: w263 -> [_ w300]
            tunnel: [w279 w299] -> w257
            tunnel: [w278 w298] -> w256
            tunnel: [w277 w297] -> w255
            tunnel: [w276 w296] -> w254
            tunnel: w262 -> [w286 _]
            frame False {
              # "Decrement Score by"
              n126 = Subtract(x=w295, y=w291) -> (x-y=w289:dbl)
              n127 = Add(x=w291, y=w294) -> (x+y=w288:dbl)
              n128 = Subtract(x=w293, y=w292) -> (x-y=w290:dbl)
              n129 = call "IMAQ Convert ROI to Rectangle"("ROI Descriptor"=w286) -> ("Rectangle"=w287:T16)  [unwired: 8 in, 1 out]
              n130 = Unbundle By Name(w287) -> ("Left"=w283:i32, "Top"=w282:i32, "Right"=w281:i32, "Bottom"=w280:i32)
              n131 = Subtract(x=w283, y="Main ROI Decay\nper Fail (Horiztonal)") -> (x-y=w279:i32)
              n132 = Add(x=w281, y="Main ROI Decay\nper Fail (Horiztonal)") -> (x+y=w277:i32)
              n133 = Add(x=w280, y="Main ROI Decay\nper Fail (Vertical)") -> (x+y=w276:i32)
              n134 = Subtract(x=w282, y="Main ROI Decay\nper Fail (Vertical)") -> (x-y=w278:i32)
            }
            frame True {
              # "Scale / Score"
              # "Main ROI"
              # "Horizontal Scale \n(smaller number = smaller ROI)"
              n135 = Subtract(x=w317, y=w314) -> (x-y=w313:dbl)
              n136 = Subtract(x=w316, y=w315) -> (x-y=w312:dbl)
              n137 = Add(x=w315, y=w316) -> (x+y=w311:dbl)
              n138 = Array To Cluster(array=w300) -> (cluster=w310:T13)
              n139 = Unbundle By Name(w310) -> ("Matches (Geometric Matching 1)[0].Position.x"=w304:sgl, "Matches (Geometric Matching 1)[0].Position.y"=w306:sgl, "Matches (Geometric Matching 1)[0].Scale"=w305:sgl)
              n140 = Divide(x=w305, y=w302) -> (x/y=w307:sgl)
              n141 = Multiply(x=w305, y=w301) -> (x*y=w309:sgl)
              n142 = Divide(x=w309, y=sgl 2.0) -> (x/y=w303:sgl)
              n143 = Add(x=w306, y=w307) -> (x+y=w296:sgl)
              n144 = Subtract(x=w306, y=w307) -> (x-y=w298:sgl)
              n145 = Subtract(x=w304, y=w303) -> (x-y=w299:sgl)
              n146 = Add(x=w303, y=w304) -> (x+y=w297:sgl)
            }
          }
          n147 = call "Bound_RO_R_R0I.vi"("Bottom Right - Y"=w254, "Right - X"=w255, "Top Left - Y"=w256, "Top  Left - x"=w257) -> ("ROI Descriptor"=w258:T3)  [unwired: 7 in]
        }
      }
      "Next Main ROI Descriptor" <- w40
      n148 = And(x="Startup Flag", y=w82) -> (x .and. y?=w85:bool)
      n149 = case shown="True" w85 {
        tunnel: "Startup Flag" -> [w231 _]
        tunnel: [w231 FALSE] -> w84
        frame False {
        }
        frame True {
        }
      }
      "Startup Flag - out" <- w84
      n150 = Less?(x=w88, y="Absolute\nMinimum Score") -> (x < y?=w92:bool)
      n151 = Less?(x=w53, y="Absolute\nMinimum Scale") -> (x < y?=w56:bool)
      n152 = Greater?(x=w54, y="Absolute\nMaximum Scale") -> (0:w51:bool)
      n153 = Greater?(x=w53, y=w54) -> (0:w57:bool)
      n154 = Less?(x=w54, y=w53) -> (x < y?=w52:bool)
      n155 = Select(t="Absolute\nMinimum Score", s=w92, f=w88) -> (s? t:f=w94:dbl)
      "New Min Score" <- w94
      n156 = Or(x=w56, y=w57) -> (x .or. y?=w58:bool)
      n157 = Or(x=w51, y=w52) -> (x .or. y?=w55:bool)
      n158 = Select(t="Absolute\nMinimum Scale", s=w58, f=w53) -> (s? t:f=w72:dbl)
      "New Low Scale" <- w72
      n159 = Select(t="Absolute\nMaximum Scale", s=w55, f=w54) -> (s? t:f=w73:dbl)
      "New high Scale" <- w73
      n160 = Bundle("index"=w90, "Min Scale"=w72, "Max Scale"=w73) -> (w89:T17)  [unwired: 1 in]
      n161 = Replace Array Subset(array=w87, new element=w89, index=w90) -> (w91:T8[])
      n162 = call "IMAQ Overlay ROI"("ROI Descriptor"=w40, "Image"=w71) -> ("Image Out"=→"Right Image 2":T6)  [unwired: 8 in, 1 out]
      n163 = Bundle By Name(cluster="Current Settings", "Range Settings"=w91, "Minimum Match Score"=w94) -> (→"New Settings":T9)
    }
  }
